vi "GT Set Auto Focus Aux Prm.vi"(6 "chanel":i16, 7 "limitKd":dbl, 8 "error in (no error)":errorcluster caption="错误输入（无错误）", 9 "kd":dbl, 10 "kf":dbl, 11 "cardNum":i16) -> (0 "error out":errorcluster caption="错误输出", 3 "function return":i16)   [LabVIEW 2014, in "gts.lvlib"]
doc: "GT_API GT_SetAutoFocusAuxPrm(short cardNum,double kf,double kd,double limitKd,short chanel);"
uses:
  gts.lvlib
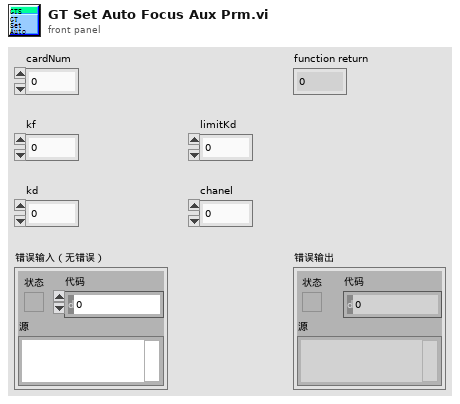
[diagram p1: front panel]
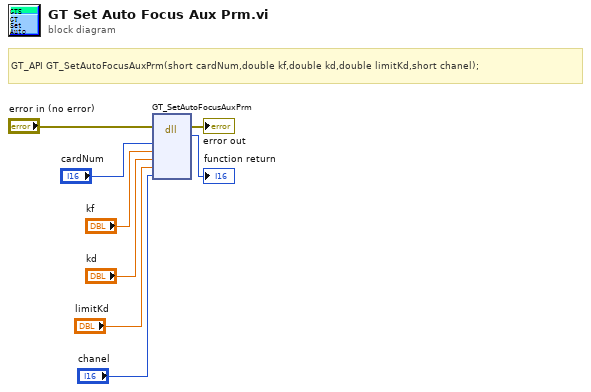
[diagram p0: block diagram]
diagram:
  # "GT_API GT_SetAutoFocusAuxPrm(short cardNum,double kf,double kd,double limitKd,short chanel);"
  n1 = dll-call lib="PTH2habs D固高科技资料GTS控制卡GTS卡18年上半年资料dllVC32bit\nmulti_cardgts.*" fn="GT_SetAutoFocusAuxPrm"(error in="error in (no error)", "cardNum"="cardNum", "kf"="kf", "kd"="kd", "limitKd"="limitKd", "chanel"="chanel") -> (error out=→"error out":errorcluster, →"function return":i16)  [unwired: 7 in, 1 out]
